vi "gridarray.vi"(0 "X Start":dbl, 1 "Y Start":dbl, 2 "Z Start":dbl, 3 "Theta End":dbl, 5 "X Step":dbl, 6 "Theta Step":dbl, 7 "Z End":dbl, 8 "Theta on":bool, 9 "Y Step":dbl, 11 "Theta Start":dbl, 12 "Y End":dbl, 13 "X End":dbl, 14 "Z Step":dbl) -> (4 "Array":dbl[][](array[numeric]))   [LabVIEW 2020]
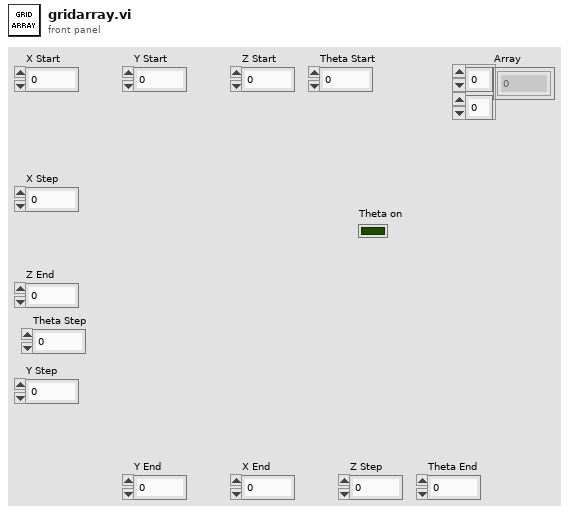
[diagram p1: front panel]
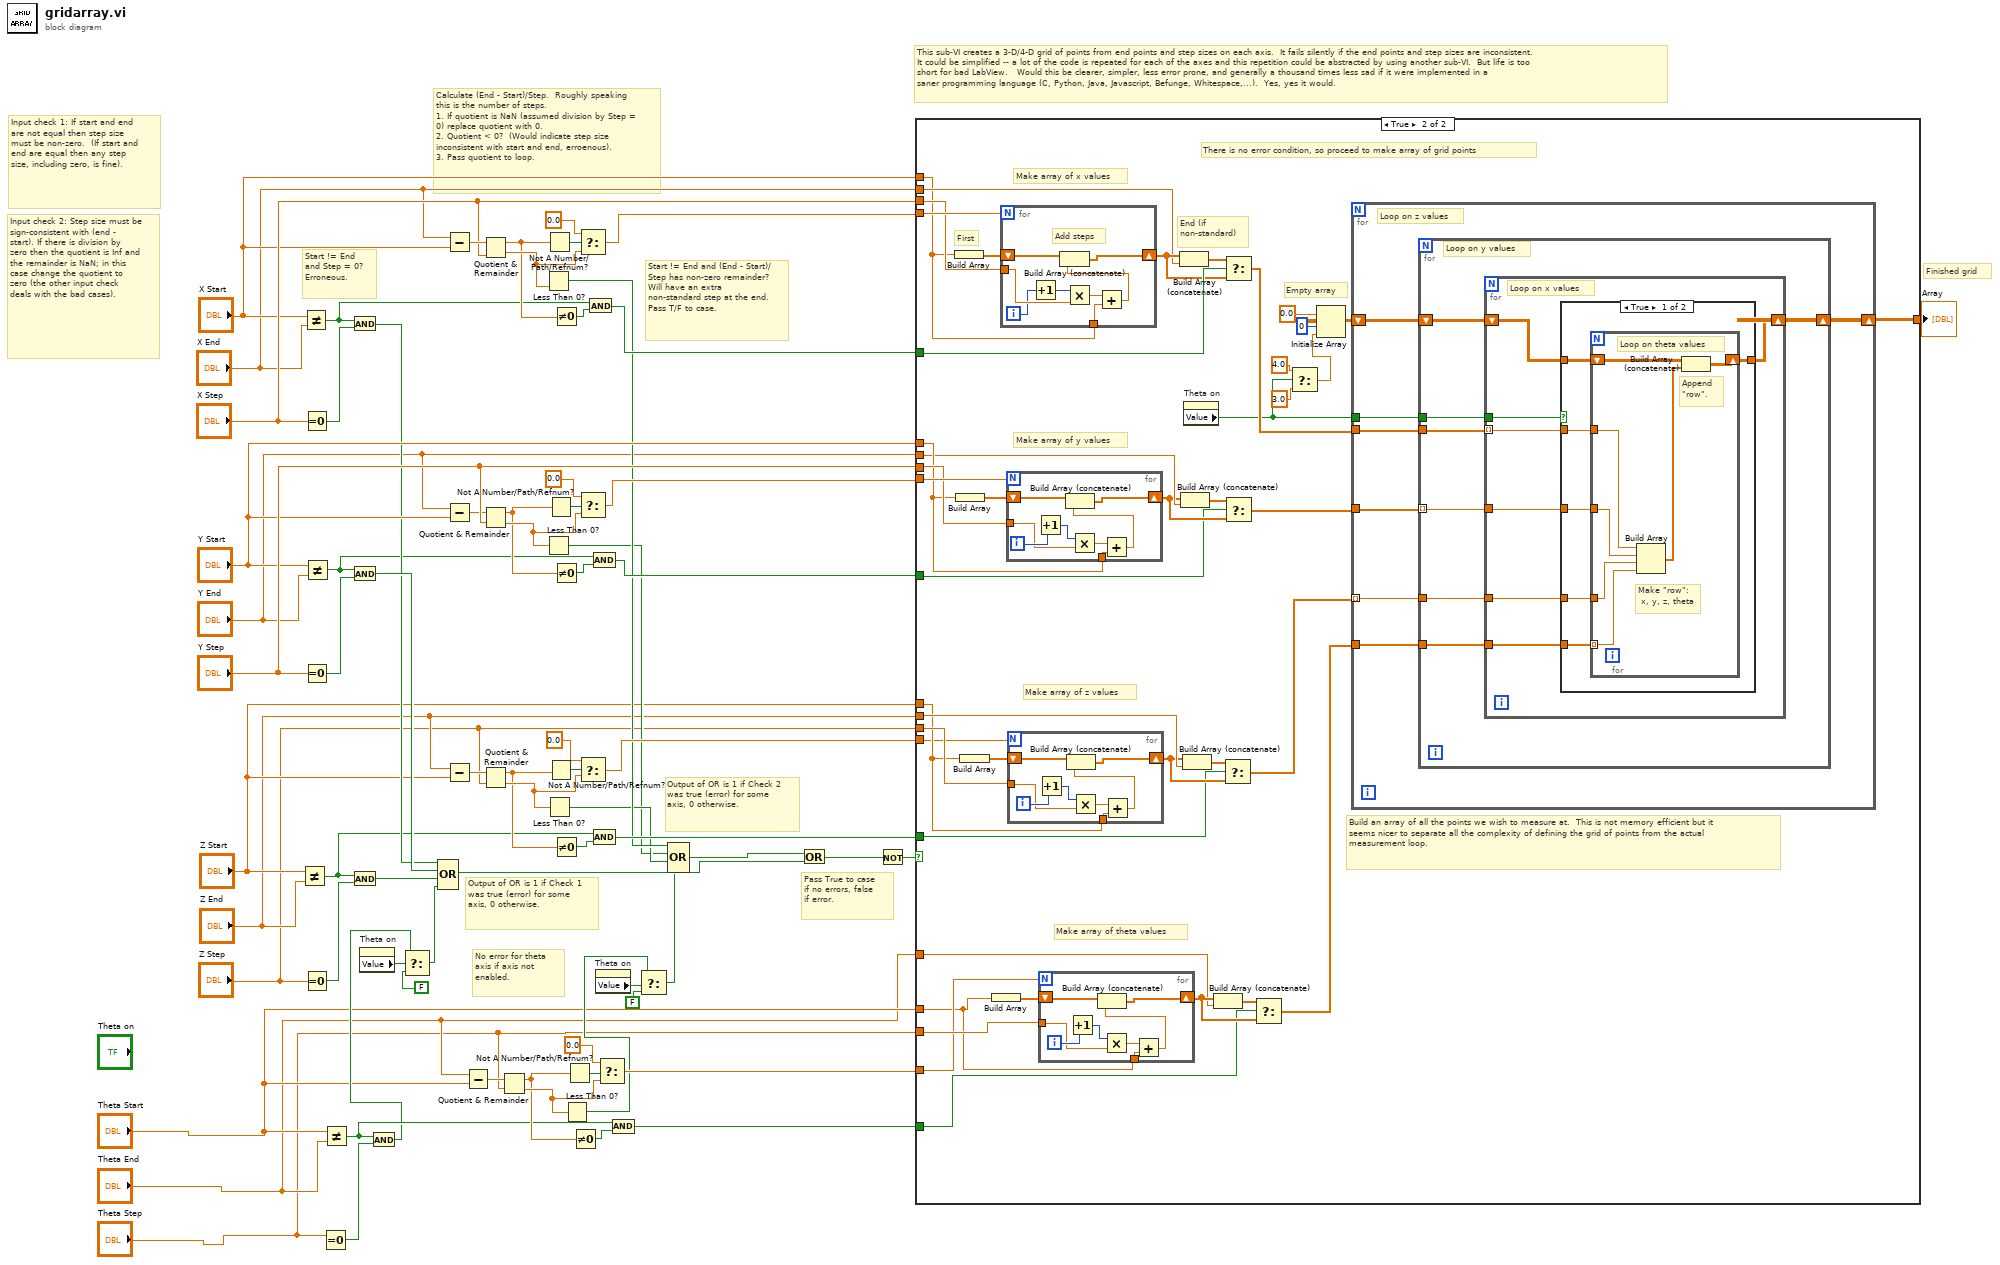
[diagram p0: block diagram]
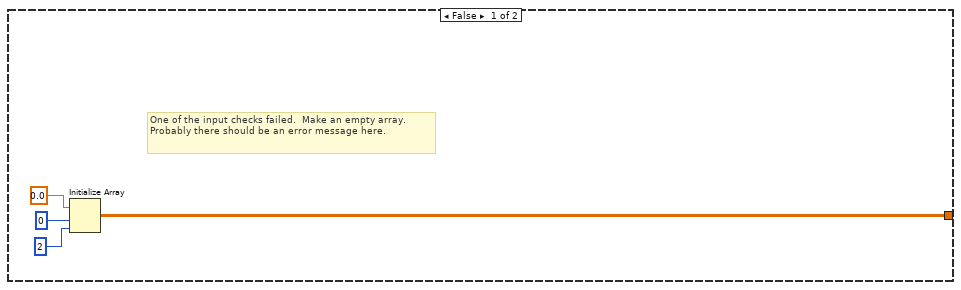
[diagram p2: hidden frame]
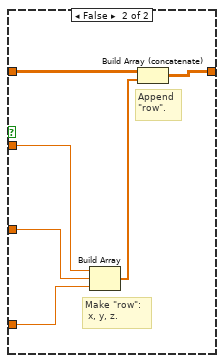
[diagram p3: hidden frame]
diagram:
  # "No error for theta axis if axis not enabled."
  # "This sub-VI creates a 3-D/4-D grid of points from end points and step sizes on each axis.  It fails silently if the end points and step sizes are inconsistent.\nIt could be simplified -- a lot of the code is repeated for each of the axes and this repetition could be abstracted by using another sub-VI.  But life is too \nshort for bad LabView.   Would this be clearer, simpler, less error prone, and generally a thousand times less sad if it were implemented in a \nsaner programming language (C, Python, Java, Javascript, Befunge, Whitespace,...).  Yes, yes it would."
  # "Finished grid"
  # "Pass True to case if no errors, false\nif error."
  # "Output of OR is 1 if Check 2 was true (error) for some axis, 0 otherwise."
  # "Output of OR is 1 if Check 1 was true (error) for some axis, 0 otherwise."
  # "Start != End and (End - Start)/Step has non-zero remainder?  Will have an extra non-standard step at the end.  Pass T/F to case."
  # "Calculate (End - Start)/Step.  Roughly speaking this is the number of steps. \n1. If quotient is NaN (assumed division by Step = 0) replace quotient with 0.  \n2. Quotient < 0?  (Would indicate step size inconsistent with start and end, erroenous). \n3. Pass quotient to loop."
  # "Start != End and Step = 0?\nErroneous."
  # "Input check 2: Step size must be sign-consistent with (end - start). If there is division by zero then the quotient is Inf and the remainder is NaN; in this case change the quotient to zero (the other input check deals with the bad cases)."
  # "Input check 1: If start and end are not equal then step size must be non-zero.  (If start and end are equal then any step size, including zero, is fine)."
  n1 = Not Equal?(x="Z Start", y="Z End") -> (x != y?=w26:bool)
  n2 = Not Equal?(x="X Start", y="X End") -> (x != y?=w49:bool)
  n3 = Equal To 0?(x="X Step") -> (x = 0?=w34:bool)
  n4 = Equal To 0?(x="Y Step") -> (x = 0?=w35:bool)
  n5 = Equal To 0?(x="Z Step") -> (x = 0?=w36:bool)
  n6 = Not Equal?(x="Y Start", y="Y End") -> (x != y?=w27:bool)
  n7 = Equal To 0?(x="Theta Step") -> (x = 0?=w16:bool)
  n8 = Not Equal?(x="Theta Start", y="Theta End") -> (x != y?=w14:bool)
  n9 = And(x=w49, y=w34) -> (x .and. y?=w37:bool)
  n10 = And(x=w27, y=w35) -> (x .and. y?=w38:bool)
  n11 = And(x=w26, y=w36) -> (x .and. y?=w39:bool)
  n12 = property on="Theta on" class="Bool (strict)"() -> ("Value"=w11:bool)  [unwired: 2 in, 2 out]
  n13 = And(x=w14, y=w16) -> (x .and. y?=w10:bool)
  n14 = Select(t=w10, s=w11, f=FALSE) -> (s? t:f=w8:bool)
  n15 = Compound Arithmetic op=OR(w37, w38, w39, w8) -> (w57:bool)
  n16 = Subtract(x="X End", y="X Start") -> (x-y=w31:dbl)
  n17 = Subtract(x="Y End", y="Y Start") -> (x-y=w32:dbl)
  n18 = Subtract(x="Z End", y="Z Start") -> (x-y=w33:dbl)
  n19 = Subtract(x="Theta End", y="Theta Start") -> (x-y=w15:dbl)
  n20 = Quotient & Remainder(x=w31, y="X Step") -> (x-y*floor(x/y)=w53:dbl, floor(x/y)=w59:dbl)
  n21 = Quotient & Remainder(x=w32, y="Y Step") -> (x-y*floor(x/y)=w54:dbl, floor(x/y)=w61:dbl)
  n22 = Quotient & Remainder(x=w33, y="Z Step") -> (x-y*floor(x/y)=w62:dbl, floor(x/y)=w70:dbl)
  n23 = Quotient & Remainder(x=w15, y="Theta Step") -> (x-y*floor(x/y)=w20:dbl, floor(x/y)=w21:dbl)
  n24 = Less Than 0?(x=w59) -> (x < 0?=w42:bool)
  n25 = Less Than 0?(x=w61) -> (x < 0?=w40:bool)
  n26 = Not A Number/Path/Refnum?(number/path/refnum=w53) -> (NaN/Path/Refnum?=w43:bool)
  n27 = Less Than 0?(x=w70) -> (x < 0?=w41:bool)
  n28 = Not A Number/Path/Refnum?(number/path/refnum=w54) -> (NaN/Path/Refnum?=w45:bool)
  n29 = Not A Number/Path/Refnum?(number/path/refnum=w62) -> (NaN/Path/Refnum?=w47:bool)
  n30 = Not Equal To 0?(x=w53) -> (x != 0?=w50:bool)
  n31 = Not Equal To 0?(x=w54) -> (x != 0?=w51:bool)
  n32 = Not Equal To 0?(x=w62) -> (x != 0?=w52:bool)
  n33 = Less Than 0?(x=w21) -> (x < 0?=w5:bool)
  n34 = Not A Number/Path/Refnum?(number/path/refnum=w20) -> (NaN/Path/Refnum?=w17:bool)
  n35 = Not Equal To 0?(x=w20) -> (x != 0?=w19:bool)
  n36 = Select(t=0.0, s=w43, f=w59) -> (s? t:f=w63:dbl)
  n37 = Select(t=0.0, s=w45, f=w61) -> (s? t:f=w65:dbl)
  n38 = Select(t=0.0, s=w47, f=w70) -> (s? t:f=w68:dbl)
  n39 = And(x=w49, y=w50) -> (x .and. y?=w55:bool)
  n40 = And(x=w27, y=w51) -> (x .and. y?=w67:bool)
  n41 = And(x=w26, y=w52) -> (x .and. y?=w69:bool)
  n42 = property on="Theta on" class="Bool (strict)"() -> ("Value"=w6:bool)  [unwired: 2 in, 2 out]
  n43 = Select(t=0.0, s=w17, f=w21) -> (s? t:f=w13:dbl)
  n44 = And(x=w14, y=w19) -> (x .and. y?=w12:bool)
  n45 = Select(t=w5, s=w6, f=FALSE) -> (s? t:f=w4:bool)
  n46 = Compound Arithmetic op=OR(w42, w40, w41, w4) -> (w56:bool)
  n47 = Or(x=w56, y=w57) -> (x .or. y?=w60:bool)
  n48 = Not(x=w60) -> (.not. x?=w58:bool)
  n49 = case shown="True" w58 {
    tunnel: "X Start" -> [_ w89]
    tunnel: w63 -> [_ w119]
    tunnel: "X Step" -> [_ w117]
    tunnel: w55 -> [_ w116]
    tunnel: "X End" -> [_ w114]
    tunnel: "Y Start" -> [_ w108]
    tunnel: w65 -> [_ w110]
    tunnel: "Y Step" -> [_ w109]
    tunnel: "Y End" -> [_ w107]
    tunnel: w67 -> [_ w105]
    tunnel: "Z Start" -> [_ w101]
    tunnel: "Z End" -> [_ w103]
    tunnel: "Z Step" -> [_ w102]
    tunnel: w68 -> [_ w98]
    tunnel: w69 -> [_ w97]
    tunnel: [w73 w90] -> w71
    tunnel: "Theta Start" -> [_ w81]
    tunnel: "Theta End" -> [_ w85]
    tunnel: "Theta Step" -> [_ w84]
    tunnel: w13 -> [_ w83]
    tunnel: w12 -> [_ w82]
    frame False {
      # "One of the input checks failed.  Make an empty array.  Probably there should be an error message here."
      n50 = Initialize Array(0.0 ("element"), 0 ("dimension size"), 2 ("dimension size")) -> (w73:dbl[][])
    }
    frame True {
      # "Make array of theta values"
      # "Build an array of all the points we wish to measure at.  This is not memory efficient but it seems nicer to separate all the complexity of defining the grid of points from the actual measurement loop."
      # "Empty array"
      # "Make array of z values"
      # "Make array of y values"
      # "There is no error condition, so proceed to make array of grid points"
      # "End (if non-standard)"
      # "First"
      # "Make array of x values"
      n51 = Build Array(w89) -> (w118:dbl[])
      n52 = Build Array(w108) -> (w111:dbl[])
      n53 = Build Array(w101) -> (w104:dbl[])
      n54 = Build Array(w81) -> (w88:dbl[])
      n55 = for {
        N: w119 -> [_]
        tunnel: w117 -> [w188]
        tunnel: w89 -> [w186]
        shift-right: [w185] -> w115
        shift-left: w118 -> [w191]
        i -> [w187]
        # "Add steps"
        n56 = Increment(x=w187) -> (x+1=w190:i32)
        n57 = Multiply(x=w190, y=w188) -> (x*y=w189:dbl)
        n58 = Add(x=w189, y=w186) -> (x+y=w184:dbl)
        n59 = Build Array (concatenate)(w191, w184) -> (w185:dbl[])
      }
      n60 = for {
        N: w110 -> [_]
        shift-right: [w179] -> w106
        shift-left: w111 -> [w183]
        tunnel: w109 -> [w177]
        tunnel: w108 -> [w176]
        i -> [w180]
        n61 = Increment(x=w180) -> (x+1=w182:i32)
        n62 = Multiply(x=w182, y=w177) -> (x*y=w181:dbl)
        n63 = Add(x=w181, y=w176) -> (x+y=w178:dbl)
        n64 = Build Array (concatenate)(w183, w178) -> (w179:dbl[])
      }
      n65 = for {
        N: w98 -> [_]
        shift-right: [w171] -> w99
        shift-left: w104 -> [w175]
        tunnel: w102 -> [w169]
        tunnel: w101 -> [w168]
        i -> [w172]
        n66 = Increment(x=w172) -> (x+1=w174:i32)
        n67 = Multiply(x=w174, y=w169) -> (x*y=w173:dbl)
        n68 = Add(x=w173, y=w168) -> (x+y=w170:dbl)
        n69 = Build Array (concatenate)(w175, w170) -> (w171:dbl[])
      }
      n70 = for {
        N: w83 -> [_]
        shift-right: [w123] -> w86
        shift-left: w88 -> [w127]
        tunnel: w84 -> [w121]
        tunnel: w81 -> [w120]
        i -> [w124]
        n71 = Increment(x=w124) -> (x+1=w126:i32)
        n72 = Multiply(x=w126, y=w121) -> (x*y=w125:dbl)
        n73 = Add(x=w125, y=w120) -> (x+y=w122:dbl)
        n74 = Build Array (concatenate)(w127, w122) -> (w123:dbl[])
      }
      n75 = Build Array (concatenate)(w115, w114) -> (w113:dbl[])
      n76 = Build Array (concatenate)(w106, w107) -> (w112:dbl[])
      n77 = Build Array (concatenate)(w99, w103) -> (w100:dbl[])
      n78 = property on="Theta on" class="Bool (strict)"() -> ("Value"=w77:bool)  [unwired: 2 in, 2 out]
      n79 = Build Array (concatenate)(w86, w85) -> (w87:dbl[])
      n80 = Select(t=w100, s=w97, f=w99) -> (s? t:f=w91:dbl[])
      n81 = Select(t=w113, s=w116, f=w115) -> (s? t:f=w93:dbl[])
      n82 = Select(t=w112, s=w105, f=w106) -> (s? t:f=w92:dbl[])
      n83 = Select(t=w87, s=w82, f=w86) -> (s? t:f=w76:dbl[])
      n84 = Select(t=4.0, s=w77, f=3.0) -> (s? t:f=w78:dbl)
      n85 = Initialize Array(0.0 ("element"), 0 ("dimension size"), w78) -> (w94:dbl[][])
      n86 = for {
        shift-right: [w130] -> w90
        shift-left: w94 -> [w134]
        tunnel: w93 -> [w133]
        tunnel: w92 -> [w132]
        tunnel: w91 -> [w131] mode=indexing
        tunnel: w77 -> [w129]
        tunnel: w76 -> [w128]
        # "Loop on z values"
        n87 = for {
          shift-right: [w137] -> w130
          shift-left: w134 -> [w141]
          tunnel: w133 -> [w140]
          tunnel: w132 -> [w139] mode=indexing
          tunnel: w131 -> [w138]
          tunnel: w129 -> [w136]
          tunnel: w128 -> [w135]
          # "Loop on y values"
          n88 = for {
            tunnel: w140 -> [w145] mode=indexing
            tunnel: w139 -> [w144]
            tunnel: w138 -> [w143]
            shift-right: [w146] -> w137
            shift-left: w141 -> [w147]
            tunnel: w136 -> [w148]
            tunnel: w135 -> [w142]
            # "Loop on x values"
            n89 = case shown="True" w148 {
              tunnel: w147 -> [w154 w167]
              tunnel: [w153 w166] -> w146
              tunnel: w145 -> [w152 w165]
              tunnel: w144 -> [w151 w164]
              tunnel: w143 -> [w150 w163]
              tunnel: w142 -> [w149 _]
              frame True {
                n90 = for {
                  tunnel: w152 -> [w158]
                  tunnel: w151 -> [w157]
                  tunnel: w150 -> [w156]
                  shift-right: [w159] -> w153
                  shift-left: w154 -> [w160]
                  tunnel: w149 -> [w155] mode=indexing
                  # "Make \"row\":\n x, y, z, theta"
                  # "Append\n\"row\"."
                  # "Loop on theta values"
                  n91 = Build Array(w158, w157, w156, w155) -> (w161:dbl[])
                  n92 = Build Array (concatenate)(w160, w161) -> (w159:dbl[][])
                }
              }
              frame False {
                # "Make \"row\":\n x, y, z."
                # "Append\n\"row\"."
                n93 = Build Array(w165, w164, w163) -> (w162:dbl[])
                n94 = Build Array (concatenate)(w167, w162) -> (w166:dbl[][])
              }
            }
          }
        }
      }
    }
  }
  "Array" <- w71
